vi "GDX_Meter.vi"() -> ()   [LabVIEW 2019]
panel:
  out "Units 5":string
  out "Units 4":string
  out "Units 3":string
  out "Units 2":string
  out "Units 1":string
  out "Ch Description 5":string
  out "Ch Description 4":string
  out "Ch Description 3":string
  out "Ch Description 2":string
  out "Ch Description 1":string
  out "Numeric 5":dbl caption="Numeric 3" format="%.3g"
  out "Numeric 4":dbl caption="m/s²" format="%.3g"
  out "Data":dbl[](array[numeric])
  out "Numeric 3":dbl caption="m/s²" format="%.3g"
  out "Numeric 2":dbl caption="m/s²" format="%.3g"
  out "Numeric 1":dbl caption="N" format="%.3g"
  in  "stop":bool
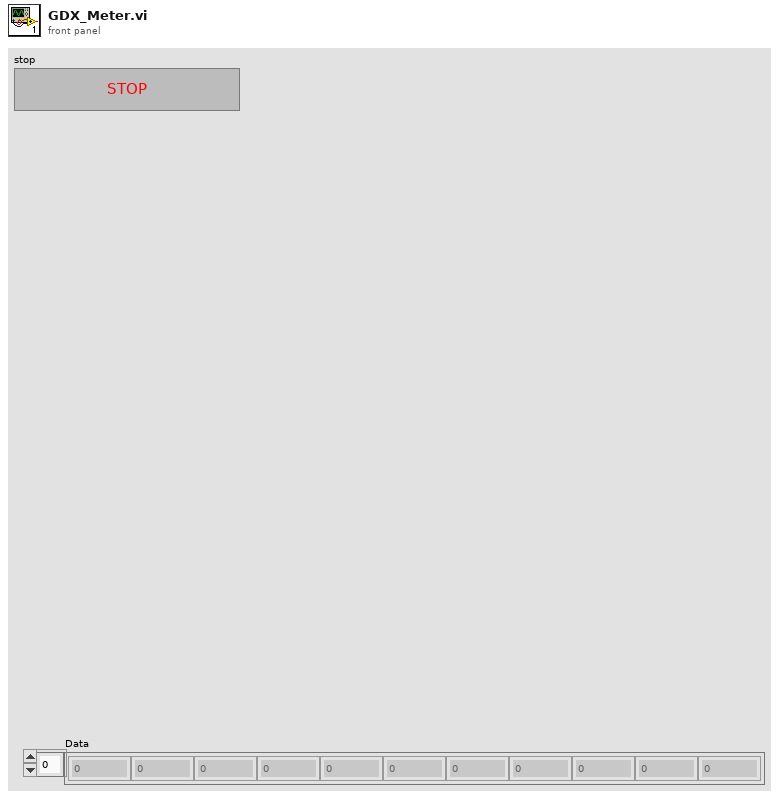
[diagram p1: front panel]
types:
  T1 = enum16{"Activate from Dialog Popup", "Activate All Channels", "Input On/Off Array", "Input Channel  Mask", "Burn Sensor Default Channels"}
  T2 = enum16{"Set Rate from Dialog Popup", "Default 1 Sample/Sec", "Input Sample Rate"}
  T3 = typedef "D2PIO_D2PIOCluster.ctl" = cluster{"Library Handle":i64, "Device List Handle":i64, "BT Device Handles":i64[], "USB Device Handles":i64[], "BT+USB Device Handles":i64[], "Measurement Tick":dbl[], "Ch Availability Mask":u32[]}
  T4 = typedef "D2PIO_ChannelInfoCluster.ctl" = cluster{"Channel":i8, "Ch is Active":bool, "Channel ID":u32, "Channel Description":string, "Channel Unit":string}[]
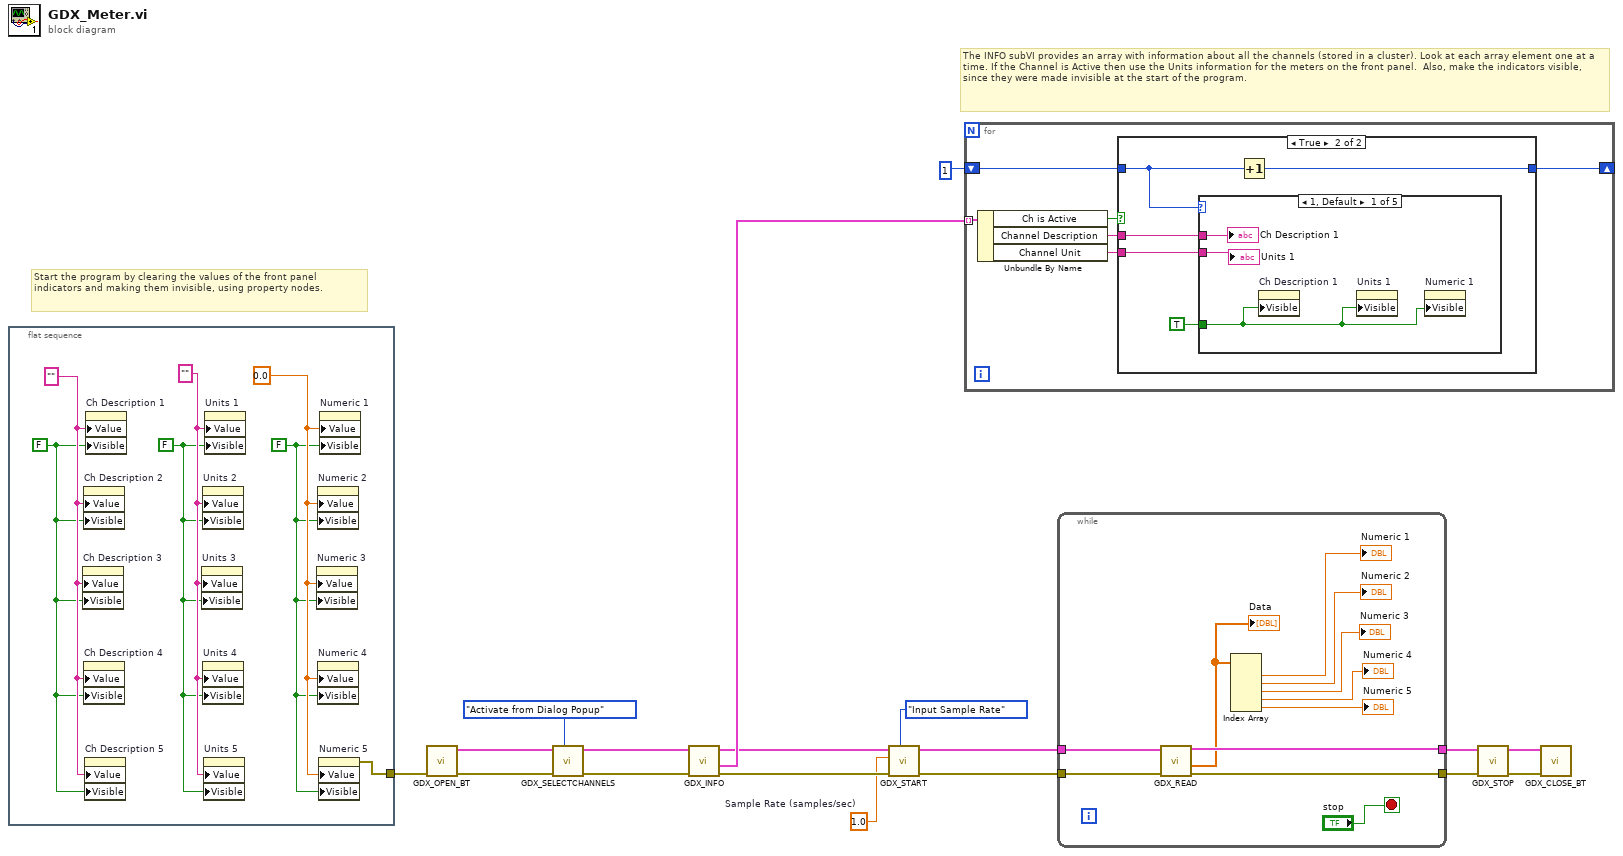
[diagram p0: block diagram]
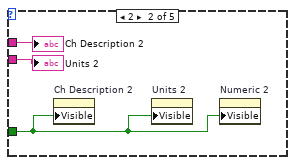
[diagram p3: hidden frame]
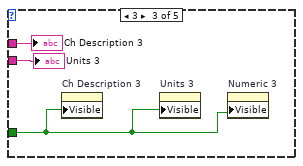
[diagram p4: hidden frame]
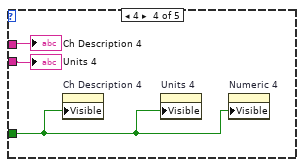
[diagram p5: hidden frame]
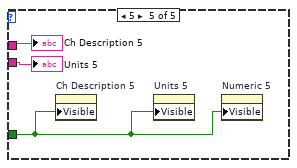
[diagram p6: hidden frame]
diagram:
  w2 = 1.0  # Sample Rate (samples/sec)
  # "Start the program by clearing the values of the front panel indicators and making them invisible, using property nodes."
  # "The INFO subVI provides an array with information about all the channels (stored in a cluster). Look at each array element one at a time. If the Channel is Active then use the Units information for the meters on the front panel.  Also, make the indicators visible, since they were made invisible at the start of the program."
  n1 = flat-sequence {
    tunnel: [w22] -> w1
    frame #0 {
      w19 = FALSE ("Visible")
      w20 = FALSE ("Visible")
      w21 = FALSE ("Visible")
      w23 = 0.0 ("Numeric 1")
      w24 = "" ("Ch Description 1")
      w25 = "" ("Ch Description 1")
      n2 = property on="Ch Description 3" class="Str"("Value"=w25, "Visible"=w21) -> ()  [unwired: 2 in, 2 out]
      n3 = property on="Ch Description 2" class="Str"("Value"=w25, "Visible"=w21) -> ()  [unwired: 2 in, 2 out]
      n4 = property on="Ch Description 4" class="Str"("Value"=w25, "Visible"=w21) -> ()  [unwired: 2 in, 2 out]
      n5 = property on="Ch Description 5" class="Str"("Value"=w25, "Visible"=w21) -> ()  [unwired: 2 in, 2 out]
      n6 = property on="Ch Description 1" class="Str"("Value"=w25, "Visible"=w21) -> ()  [unwired: 2 in, 2 out]
      n7 = property on="Units 3" class="Str"("Value"=w24, "Visible"=w20) -> ()  [unwired: 2 in, 2 out]
      n8 = property on="Units 2" class="Str"("Value"=w24, "Visible"=w20) -> ()  [unwired: 2 in, 2 out]
      n9 = property on="Units 4" class="Str"("Value"=w24, "Visible"=w20) -> ()  [unwired: 2 in, 2 out]
      n10 = property on="Units 5" class="Str"("Value"=w24, "Visible"=w20) -> ()  [unwired: 2 in, 2 out]
      n11 = property on="Units 1" class="Str"("Value"=w24, "Visible"=w20) -> ()  [unwired: 2 in, 2 out]
      n12 = property on="Numeric 3" class="DigNum (strict)"("Value"=w23, "Visible"=w19) -> ()  [unwired: 2 in, 2 out]
      n13 = property on="Numeric 2" class="DigNum (strict)"("Value"=w23, "Visible"=w19) -> ()  [unwired: 2 in, 2 out]
      n14 = property on="Numeric 4" class="DigNum (strict)"("Value"=w23, "Visible"=w19) -> ()  [unwired: 2 in, 2 out]
      n15 = property on="Numeric 5" class="DigNum (strict)"("Value"=w23, "Visible"=w19) -> (error out=w22:errorcluster)  [unwired: 2 in, 1 out]
      n16 = property on="Numeric 1" class="DigNum (strict)"("Value"=w23, "Visible"=w19) -> ()  [unwired: 2 in, 2 out]
    }
  }
  n17 = call <vilib>:"GDX_OPEN_BT.vi"("error in (no error)"=w1) -> ("error out"=w12:errorcluster, "D2PIO Cluster Out"=w13:T3)  [unwired: 9 in]
  n18 = call <vilib>:"GDX_SELECTCHANNELS.vi"("Enum"=T1."Activate from Dialog Popup", "error in (no error)"=w12, "D2PIO Cluster In"=w13) -> ("error out"=w4:errorcluster, "D2PIO Cluster Out"=w7:T3)  [unwired: 7 in]
  n19 = call <vilib>:"GDX_INFO.vi"("error in (no error)"=w4, "D2PIO Cluster In"=w7) -> ("error out"=w5:errorcluster, "Array of Channel Info Cluster"=w8:T4, "D2PIO Cluster Out"=w6:T3)  [unwired: 4 in, 3 out]
  n20 = call <vilib>:"GDX_START.vi"("Enum"=T2."Input Sample Rate", "error in (no error)"=w5, "Sample Rate (samples/sec)"=w2, "D2PIO Cluster In"=w6) -> ("error out"=w18:errorcluster, "D2PIO Cluster Out"=w17:T3)  [unwired: 4 in, 2 out]
  n21 = for {
    tunnel: w8 -> [w31] mode=indexing
    shift-right: [w27] -> _
    shift-left: i8 1 ("Numeric") -> [w28]
    n22 = Unbundle By Name(w31) -> ("Ch is Active"=w29:bool, "Channel Description"=w30:string, "Channel Unit"=w26:string)
    n23 = case shown="True" w29 {
      tunnel: w30 -> [_ w37]
      tunnel: w28 -> [w32 w35]
      tunnel: [w32 w36] -> w27
      tunnel: w26 -> [_ w34]
      frame False {
      }
      frame True {
        n24 = case shown="1, Default" w35 {
          tunnel: w37 -> [w40 w43 w46 w49 w52]
          tunnel: w34 -> [w39 w42 w45 w48 w51]
          tunnel: TRUE ("Visible") -> [w38 w41 w44 w47 w50]
          frame 1, Default {
            n25 = property on="Ch Description 1" class="Str"("Visible"=w38) -> ()  [unwired: 2 in, 2 out]
            n26 = property on="Units 1" class="Str"("Visible"=w38) -> ()  [unwired: 2 in, 2 out]
            n27 = property on="Numeric 1" class="DigNum (strict)"("Visible"=w38) -> ()  [unwired: 2 in, 2 out]
            "Units 1" <- w39
            "Ch Description 1" <- w40
          }
          frame 2 {
            n28 = property on="Ch Description 2" class="Str"("Visible"=w41) -> ()  [unwired: 2 in, 2 out]
            n29 = property on="Units 2" class="Str"("Visible"=w41) -> ()  [unwired: 2 in, 2 out]
            n30 = property on="Numeric 2" class="DigNum (strict)"("Visible"=w41) -> ()  [unwired: 2 in, 2 out]
            "Ch Description 2" <- w43
            "Units 2" <- w42
          }
          frame 3 {
            n31 = property on="Ch Description 3" class="Str"("Visible"=w44) -> ()  [unwired: 2 in, 2 out]
            n32 = property on="Units 3" class="Str"("Visible"=w44) -> ()  [unwired: 2 in, 2 out]
            n33 = property on="Numeric 3" class="DigNum (strict)"("Visible"=w44) -> ()  [unwired: 2 in, 2 out]
            "Ch Description 3" <- w46
            "Units 3" <- w45
          }
          frame 4 {
            n34 = property on="Ch Description 4" class="Str"("Visible"=w47) -> ()  [unwired: 2 in, 2 out]
            n35 = property on="Units 4" class="Str"("Visible"=w47) -> ()  [unwired: 2 in, 2 out]
            n36 = property on="Numeric 4" class="DigNum (strict)"("Visible"=w47) -> ()  [unwired: 2 in, 2 out]
            "Ch Description 4" <- w49
            "Units 4" <- w48
          }
          frame 5 {
            n37 = property on="Ch Description 5" class="Str"("Visible"=w50) -> ()  [unwired: 2 in, 2 out]
            n38 = property on="Units 5" class="Str"("Visible"=w50) -> ()  [unwired: 2 in, 2 out]
            n39 = property on="Numeric 5" class="DigNum (strict)"("Visible"=w50) -> ()  [unwired: 2 in, 2 out]
            "Ch Description 5" <- w52
            "Units 5" <- w51
          }
        }
        n40 = Increment(x=w35) -> (x+1=w36:i8)
      }
    }
  }
  n41 = while {
    tunnel: w18 -> [w63]
    tunnel: w17 -> [w61]
    tunnel: [w59] -> w16
    tunnel: [w60] -> w11
    stop <- "stop" stop-if-true
    n42 = call <vilib>:"GDX_READ.vi"("error in (no error)"=w63, "D2PIO Cluster In"=w61) -> ("error out"=w60:errorcluster, "Data"=w58:dbl[], "D2PIO Cluster Out"=w59:T3)  [unwired: 4 in, 3 out]
    "Data" <- w58
    n43 = Index Array(array=w58) -> (element #1=→"Numeric 1":dbl, element #2=→"Numeric 2":dbl, element #3=→"Numeric 3":dbl, element #4=→"Numeric 4":dbl, element #5=→"Numeric 5":dbl)  [unwired: 5 in]
  }
  n44 = call <vilib>:"GDX_STOP.vi"("error in (no error)"=w11, "D2PIO Cluster In"=w16) -> ("error out"=w14:errorcluster, "D2PIO Cluster Out"=w15:T3)  [unwired: 8 in]
  n45 = call <vilib>:"GDX_CLOSE_BT.vi"("error in (no error)"=w14, "D2PIO Cluster In"=w15) -> ()  [unwired: 8 in, 2 out]
